vi "average last x days data.vi"(1 "last x days":i32, 2 "Array":i32[](array[numeric])) -> (0 "avg last x days":dbl)   [LabVIEW 2019]
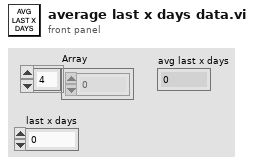
[diagram p1: front panel]
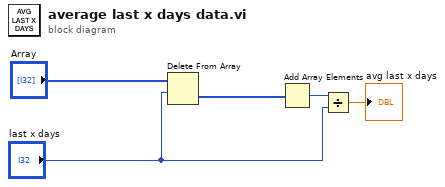
[diagram p0: block diagram]
diagram:
  n1 = Delete From Array(array="Array", length="last x days") -> (deleted portion=w4:i32[])  [unwired: 1 in, 1 out]
  n2 = Add Array Elements(numeric array=w4) -> (sum=w3:i32)
  n3 = Divide(x=w3, y="last x days") -> (x/y=→"avg last x days":dbl)
